vi "Read Color Grade Hit Ranges.vi"(8 "error in (no error)":errorcluster, 11 "VISA resource name":refnum<visa-resource-name>) -> (0 "error out":errorcluster, 2 "Color Grade Hit Ranges":i32[][](array[numeric]), 3 "VISA resource name out":refnum<visa-resource-name>)   [LabVIEW 2015, in "Agilent 2000 3000 X-Series.lvlib"]
doc: "Returns a 2-D array of the hit ranges for each color bin. The first column is the lower limits for the hit ranges and the second column is the upper limits.\n\n<b>Note:</b>\nThis VI is specific to the 6000-X Series oscilloscopes. These features are not available on other models."
uses:
  <instrlib>/Agilent 2000 3000 X-Series/Agilent 2000 3000 X-Series.lvlib
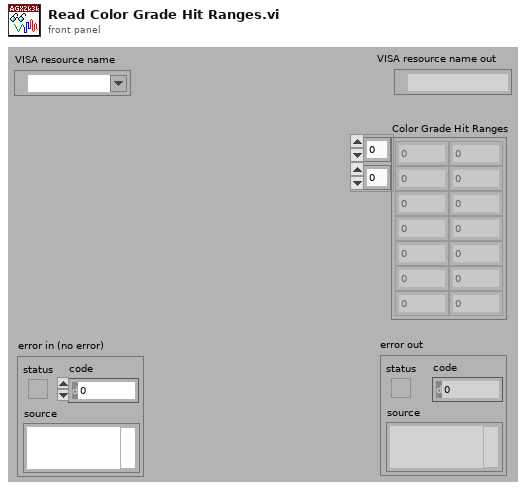
[diagram p1: front panel]
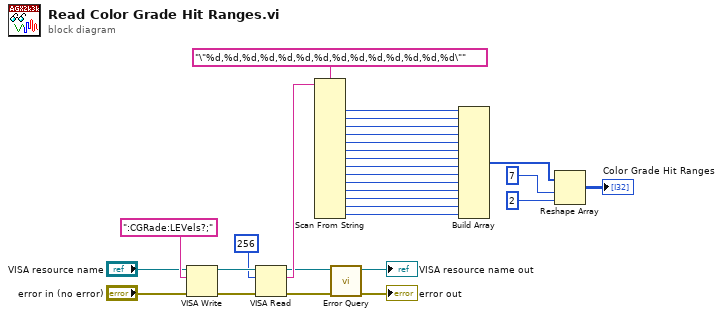
[diagram p0: block diagram]
diagram:
  n1 = VISA Write(VISA resource name="VISA resource name", write buffer=":CGRade:LEVels?;", error in (no error)="error in (no error)") -> (VISA resource name out=w27:refnum<visa-resource-name>, error out=w26:errorcluster)  [unwired: 1 out]
  n2 = VISA Read(VISA resource name=w27, byte count=u32 256, error in (no error)=w26) -> (VISA resource name out=w4:refnum<visa-resource-name>, read buffer=w24:string, error out=w3:errorcluster)  [unwired: 1 out]
  n3 = Scan From String(format string="\"%d,%d,%d,%d,%d,%d,%d,%d,%d,%d,%d,%d,%d,%d\"", input string=w24) -> (output 1=w22:i32, output 2=w21:i32, output 3=w20:i32, output 4=w19:i32, output 5=w18:i32, output 6=w17:i32, output 7=w16:i32, output 8=w15:i32, output 9=w14:i32, output 10=w13:i32, output 11=w12:i32, output 12=w11:i32, output 13=w10:i32, output 14=w9:i32)  [unwired: 16 in, 3 out]
  n4 = call <instrlib>:"Error Query.vi"("error in (no error)"=w3, "VISA resource name"=w4) -> ("error out"=→"error out":errorcluster, "VISA resource name out"=→"VISA resource name out":refnum<visa-resource-name>)  [unwired: 6 in, 2 out]
  n5 = Build Array(w22, w21, w20, w19, w18, w17, w16, w15, w14, w13, w12, w11, w10, w9) -> (w6:i32[])
  n6 = Reshape Array(w6, 7 ("dimension size"), 2 ("dimension size")) -> (→"Color Grade Hit Ranges":i32[][])
